vi "ukol 1.vi"() -> ()   [LabVIEW 2023]
uses:
  <vilib>/measure/maspectr.llb/FFT Spectrum (Mag-Phase) for 1 Chan.vi
  <vilib>/addons/Digital Filter Design/Process.llb/DFD Filtering (Wfm).vi
  <vilib>/addons/Digital Filter Design/NI_DigFilterLicensed.lvlib
  <vilib>/measure/NI_MAPro.lvlib
panel:
  out "Waveform Graph 6":waveform(dbl)[](graph)
  out "Waveform Graph 5":waveform(dbl)[](graph)
  out "Waveform Graph 4":waveform(dbl)[](graph)
  out "Waveform Graph 3":cluster{"f0":dbl, "df":dbl, "magnitude":dbl[]}[](graph)
  out "Waveform Graph 2":cluster{"f0":dbl, "df":dbl, "magnitude":dbl[]}[](graph)
  out "Waveform Graph":cluster{"f0":dbl, "df":dbl, "magnitude":dbl[]}[](graph)
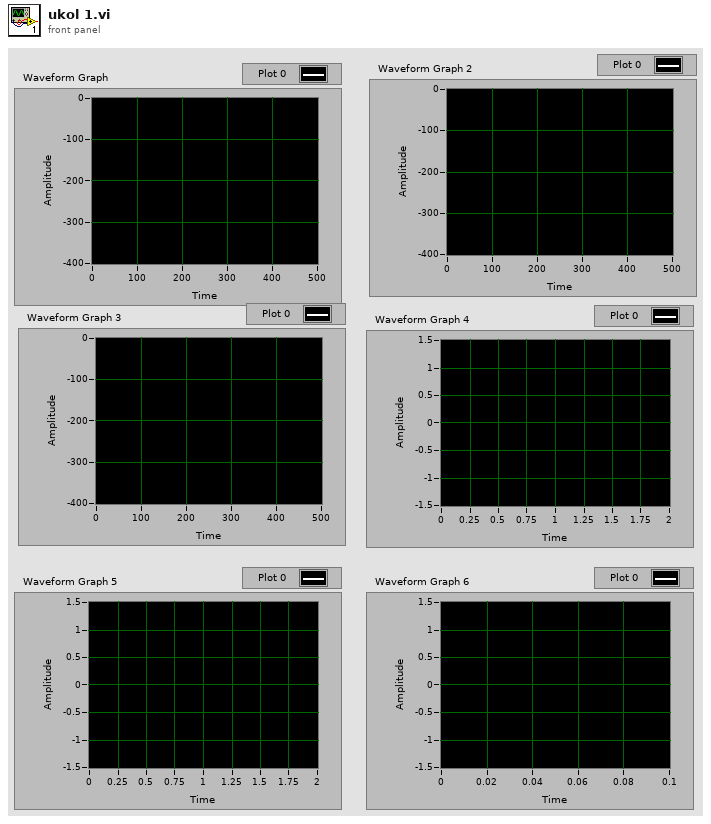
[diagram p1: front panel]
types:
  T1 = typedef "NI_DigFilterLicensed.lvlib/DFD Filter Obj.ctl" = cluster{"mSRate_Fs":dbl, "mSRate_Version":string, "mSRate_Comments":string, "mSRate_OrgCoef":T2, "mSRate_CurCoef":T2, "mSRate_Quantized?":bool, "mSRate_QCoef":T2, "mSRate_QSettings":T4[], "mSRate_Order":i32, "mSRate_Scaling":cluster{"mSRate_ScaleByPowerOf2?":bool, "mSRate_ScaleType":T6}}
  T2 = typedef "NI_DigFilterLicensed.lvlib/DFD Filter Coef.ctl" = cluster{"type":T3, "gain":dbl, "coef a (k)":dbl[], "coef b (v)":dbl[]}
  T3 = typedef "NI_DigFilterLicensed.lvlib/DFD Filter Structure Type Selector.ctl" = enum16{"Undefined", "FIR Direct Form", "FIR Direct Form Transposed", "FIR Symmetric", "FIR Antisymmetric", "IIR Direct Form I", "IIR Direct Form I Transposed", "IIR Direct Form II", "IIR Direct Form II Transposed", "IIR Cascaded Second Order Sections Form I", "IIR Cascaded Second Order Sections Form I Transposed", "IIR Cascaded Second Order Sections Form II", "IIR Cascaded Second Order Sections Form II Transposed", "Lattice Allpass (basic sections)", "Lattice Allpass (one multiplier sections)", "Lattice Allpass (normalized sections)", "Lattice AR (basic sections)", "Lattice AR (one multiplier sections)", "Lattice AR (normalized sections)", "Lattice MA (minimum phase)", "Lattice MA (maximum phase)", "Lattice ARMA (basic sections)", "Lattice ARMA (one multiplier sections)", "Lattice ARMA (normalized sections)"}
  T4 = typedef "NI_DigFilterLicensed.lvlib/dfd_Internal Quantization Settings.ctl" = cluster{"source":T5, "wl":i16, "iwl":i16, "overflow mode":enum16{"Saturation", "Wrap"}, "rounding mode":enum16{"Nearest", "Truncation"}, "signed?":bool}
  T5 = typedef "NI_DigFilterLicensed.lvlib/dfd_Internal Quantization Srcs.ctl" = u16
  T6 = typedef "NI_DigFilterLicensed.lvlib/DFD Coef Norm Type.ctl" = enum16{"No Norm", "Time Domain 1-Norm", "Time Domain 2-Norm", "Time Domain Inf-Norm"}
  T7 = cluster{"dB On (F)":bool, "unwrap phase (F)":bool, "convert to degree (F)":bool}
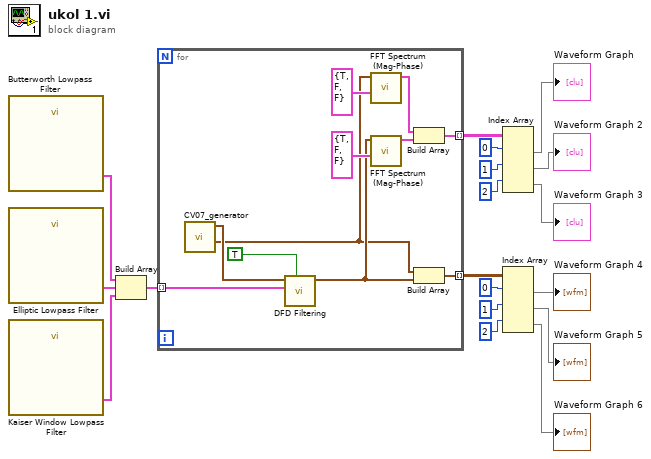
[diagram p0: block diagram]
diagram:
  n1 = call "Butterworth Lowpass Filter"() -> ("filter out"=w18:T1)  [unwired: 10 in, 1 out]
  n2 = call "Elliptic Lowpass Filter"() -> ("filter out"=w17:T1)  [unwired: 10 in, 1 out]
  n3 = call "Kaiser Window Lowpass Filter"() -> ("filter out"=w16:T1)  [unwired: 10 in, 1 out]
  n4 = Build Array(w18, w17, w16) -> (w15:T1[])
  n5 = for {
    tunnel: w15 -> [w29] mode=indexing
    tunnel: [w26] -> w14 mode=indexing
    tunnel: [w22] -> w7 mode=indexing
    n6 = call "CV07_generator.vi"() -> ("Original Sine 60 Hz"=w21:waveform(dbl), "Signal for filtration"=w23:waveform(dbl))  [unwired: 10 in]
    n7 = call-poly <vilib>:"DFD Filtering.vi"("init? (F)"=TRUE, "filter"=w29, "signal in"=w23) -> ("signal out"=w25:waveform(dbl))  [unwired: 7 in, 1 out]
    n8 = call-poly <vilib>:"FFT Spectrum (Mag-Phase).vi"("view"=T7 {"dB On (F)"=TRUE, "unwrap phase (F)"=FALSE, "convert to degree (F)"=FALSE}, "time signal"=w21) -> ("magnitude"=w19:cluster{"f0":dbl, "df":dbl, "magnitude":dbl[]})  [unwired: 5 in, 4 out]
    n9 = call-poly <vilib>:"FFT Spectrum (Mag-Phase).vi"("view"=T7 {"dB On (F)"=TRUE, "unwrap phase (F)"=FALSE, "convert to degree (F)"=FALSE}, "time signal"=w25) -> ("magnitude"=w20:cluster{"f0":dbl, "df":dbl, "magnitude":dbl[]})  [unwired: 5 in, 4 out]
    n10 = Build Array(w19, w20) -> (w22:cluster{"f0":dbl, "df":dbl, "magnitude":dbl[]}[])
    n11 = Build Array(w21, w25) -> (w26:waveform(dbl)[])
  }
  n12 = Index Array(array=w7, index (row) #1=0 ("index"), index (row) #2=1 ("index"), index (row) #3=2 ("index")) -> (element #1=→"Waveform Graph":cluster{"f0":dbl, "df":dbl, "magnitude":dbl[]}[], element #2=→"Waveform Graph 2":cluster{"f0":dbl, "df":dbl, "magnitude":dbl[]}[], element #3=→"Waveform Graph 3":cluster{"f0":dbl, "df":dbl, "magnitude":dbl[]}[])  [unwired: 3 in]
  n13 = Index Array(array=w14, index (row) #1=0 ("index"), index (row) #2=1 ("index"), index (row) #3=2 ("index")) -> (element #1=→"Waveform Graph 4":waveform(dbl)[], element #2=→"Waveform Graph 5":waveform(dbl)[], element #3=→"Waveform Graph 6":waveform(dbl)[])  [unwired: 3 in]
